vi "Main.vi"(8 "error in (no error)":errorcluster, 11 "PizzaTestDrive":refnum<class "PizzaTestDrive.lvclass">) -> (0 "error out":errorcluster, 3 "PizzaTestDrive":refnum<class "PizzaTestDrive.lvclass">)   [LabVIEW 2020, in "FactoryMethod.lvlib" / "PizzaFactoryMethod.lvlib" / "PizzaTestDrive.lvclass"]
uses:
  PizzaTestDrive.lvclass
  PizzaStore/TypeDef/PizzaId.ctl
  NYPizzaStore/NYPizzaStore.lvclass
  E:/Francesco/GitHub/Design-Patterns-GoF_-_NI-LV/Creational/FactoryMethod/Head-First_Example/PizzaFactoryMethod/PizzaStore/PizzaStore.lvclass
  ChicagoPizzaStore/ChicagoPizzaStore.lvclass
  Pizza/Pizza.lvclass
  PizzaStore/PizzaStore.lvclass
  Support/Class/ConsoleOutput.lvclass
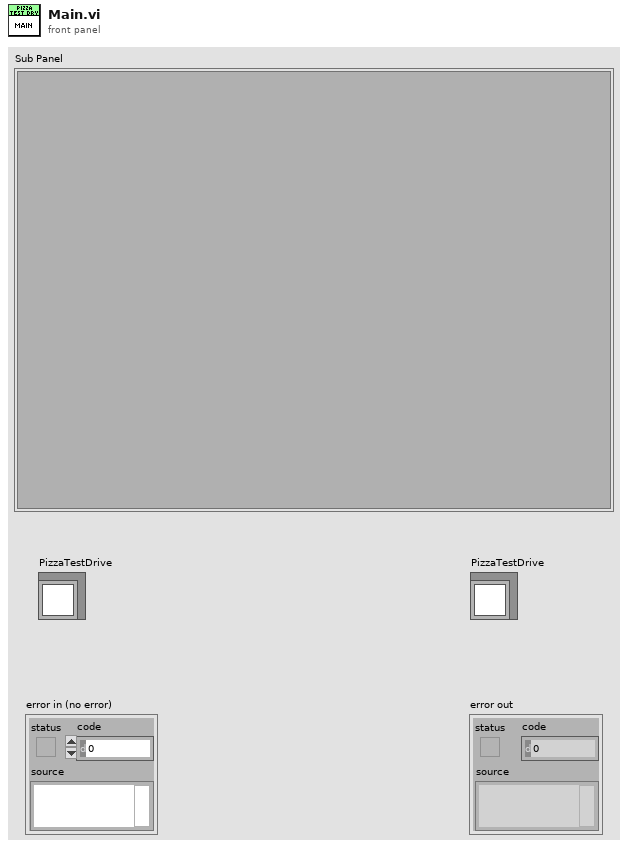
[diagram p1: front panel]
types:
  T1 = typedef "FactoryMethod.lvlib/PizzaFactoryMethod.lvlib/PizzaStore.lvclass/PizzaId.ctl" = enum16{"Cheese", "Clam", "Pepperoni", "Veggie"}
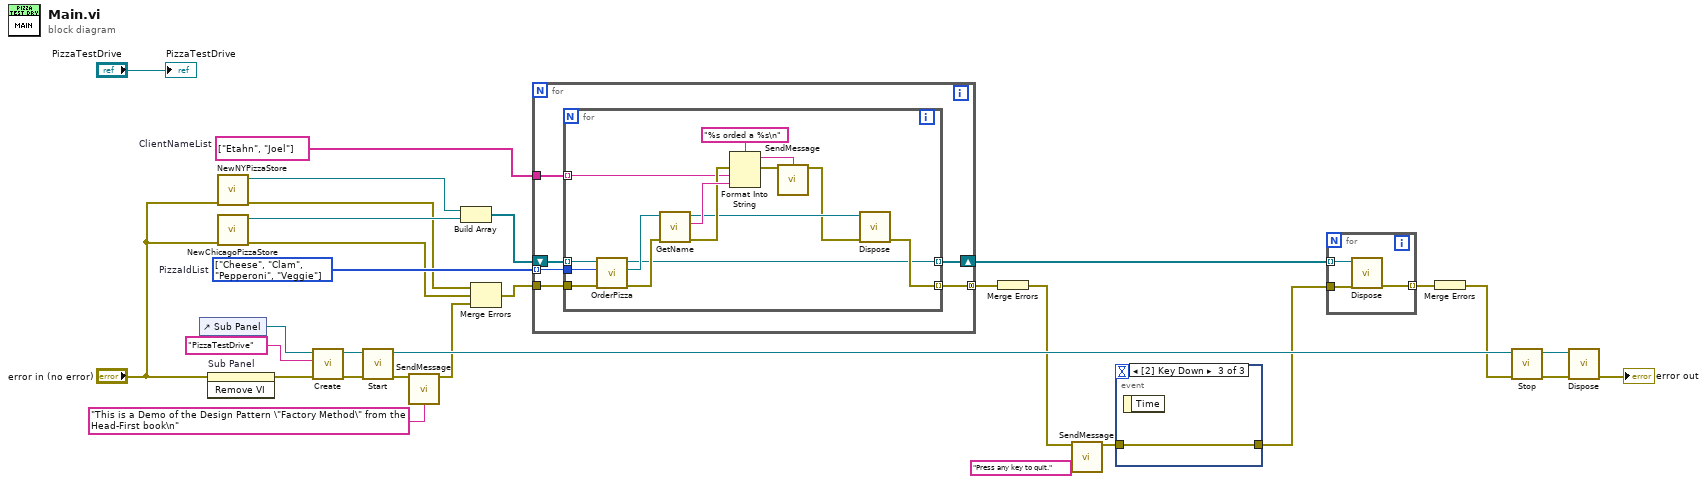
[diagram p0: block diagram]
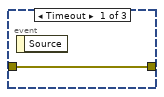
[diagram p2: hidden frame]
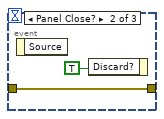
[diagram p3: hidden frame]
diagram:
  w10 = string[] ["Etahn", "Joel"]  # ClientNameList
  w12 = T1[] [enum."Cheese", enum."Clam", enum."Pepperoni", enum."Veggie"] items=["Cheese", "Clam", "Pepperoni", "Veggie"]  # PizzaIdList
  n1 = control-ref of="Sub Panel"() -> (w23:refnum<vi>)
  n2 = invoke on="Sub Panel" class="SubPnl" method="Remove VI"(error in="error in (no error)") -> (error out=w24:errorcluster)  [unwired: 2 in, 2 out]
  n3 = call "NewNYPizzaStore.vi"("error in (no error)"="error in (no error)") -> ("error out"=w4:errorcluster, "NYPizzaStore"=w7:refnum<class "NYPizzaStore.lvclass">)  [unwired: 9 in]
  n4 = call "NewChicagoPizzaStore.vi"("error in (no error)"="error in (no error)") -> ("error out"=w3:errorcluster, "ChicagoPizzaStore"=w6:refnum<class "ChicagoPizzaStore.lvclass">)  [unwired: 9 in]
  n5 = call "Create.vi"("error in (no error)"=w24, "LoggerName"="PizzaTestDrive", "SubPanelRef"=w23) -> ("error out"=w30:errorcluster, "ConsoleOutput out"=w29:refnum<class "ConsoleOutput.lvclass">)  [unwired: 7 in]
  n6 = call "Start.vi"("error in (no error)"=w30, "ConsoleOutput in"=w29) -> ("error out"=w25:errorcluster, "ConsoleOutput out"=w27:refnum<class "ConsoleOutput.lvclass">)  [unwired: 8 in]
  n7 = call "SendMessage.vi"("Message"="This is a Demo of the Design Pattern \"Factory Method\" from the Head-First book\n" ("Data"), "error in (no error)"=w25) -> ("error out"=w1:errorcluster)  [unwired: 13 in]
  n8 = Build Array(w7, w6) -> (w11:refnum<class "PizzaStore.lvclass">[])
  n9 = Merge Errors(w4, w3, w1) -> (w2:errorcluster)
  n10 = for {
    tunnel: w12 -> [w36] mode=indexing
    tunnel: w10 -> [w34]
    tunnel: [w33] -> w9 mode=concatenating
    tunnel: w2 -> [w32]
    shift-right: [w31] -> w8
    shift-left: w11 -> [w35]
    n11 = for {
      tunnel: [w44] -> w33 mode=indexing
      tunnel: w32 -> [w46]
      tunnel: w36 -> [w43]
      tunnel: w35 -> [w42] mode=indexing
      tunnel: w34 -> [w41] mode=indexing
      tunnel: [w40] -> w31 mode=indexing
      n12 = call "OrderPizza.vi"("error in (no error)"=w46, "PizzaId"=w43, "PizzaStore"=w42) -> ("error out"=w48:errorcluster, "Pizza"=w51:refnum<class "Pizza.lvclass">, "PizzaStore"=w40:refnum<class "PizzaStore.lvclass">)  [unwired: 6 in]
      n13 = call "GetName.vi"("error in (no error)"=w48, "Pizza in"=w51) -> ("error out"=w49:errorcluster, "Name"=w50:string, "Pizza out"=w45:refnum<class "Pizza.lvclass">)  [unwired: 7 in]
      n14 = Format Into String(format string="%s orded a %s\n", error in=w49, w41, w50) -> (resulting string=w38:string, error out=w39:errorcluster)  [unwired: 1 in]
      n15 = call "SendMessage.vi"("Message"=w38, "error in (no error)"=w39) -> ("error out"=w37:errorcluster)  [unwired: 13 in]
      n16 = call-dynamic "Dispose.vi"("error in (no error)"=w37, "IDisposable"=w45) -> ("error out"=w44:errorcluster)  [unwired: 9 in]
    }
  }
  n17 = Merge Errors(w9) -> (w15:errorcluster)
  n18 = call "SendMessage.vi"("Message"="Press any key to quit." ("Data"), "error in (no error)"=w15) -> ("error out"=w14:errorcluster)  [unwired: 13 in]
  n19 = event shown="[2] Key Down" {
    selector: _ -> [_ _ _]
    dyn-events: _ -> [_ _ _]
    timeout: _ -> [_ _ _]
    tunnel: w14 -> [w52 w54 w55]
    tunnel: [w52 w54 w55] -> w19
    event Timeout {
      n20 = event-data() -> ()  [unwired: 1 in, 1 out]
    }
    event Panel Close? {
      n21 = event-data() -> ()  [unwired: 1 in, 1 out]
      n22 = event-data("Discard?"=TRUE) -> ()  [unwired: 1 in, 1 out]
    }
    event Key Down {
      n23 = event-data() -> ()  [unwired: 1 in, 1 out]
    }
  }
  n24 = for {
    tunnel: w19 -> [w58]
    tunnel: [w56] -> w18 mode=indexing
    tunnel: w8 -> [w57] mode=indexing
    n25 = call-dynamic "Dispose.vi"("error in (no error)"=w58, "IDisposable"=w57) -> ("error out"=w56:errorcluster)  [unwired: 9 in]
  }
  n26 = Merge Errors(w18) -> (w17:errorcluster)
  n27 = call "Stop.vi"("error in (no error)"=w17, "ConsoleOutput in"=w27) -> ("error out"=w20:errorcluster, "ConsoleOutput out"=w28:refnum<class "ConsoleOutput.lvclass">)  [unwired: 8 in]
  n28 = call "Dispose.vi"("error in (no error)"=w20, "ConsoleOutput in"=w28) -> ("error out"=→"error out":errorcluster)  [unwired: 9 in]
  "PizzaTestDrive" <- "PizzaTestDrive"
